vi "html Table.vi"(9 "Rows cnt":u32, 10 "Table Header":string, 11 "In String Table":string[][](array[string])) -> (3 "html string out":string)   [LabVIEW 2018]
panel:
  # "HTML TABLE REPORT GENERATION"
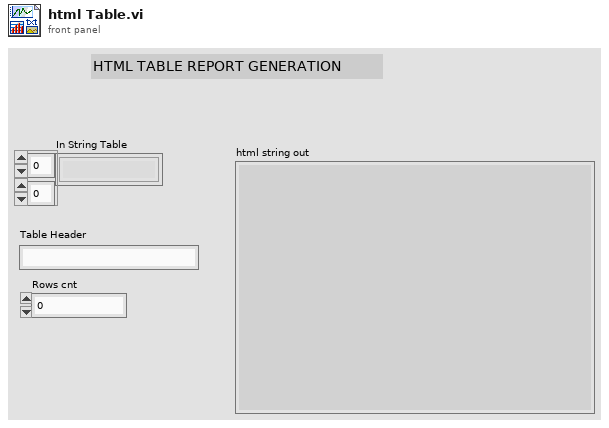
[diagram p1: front panel]
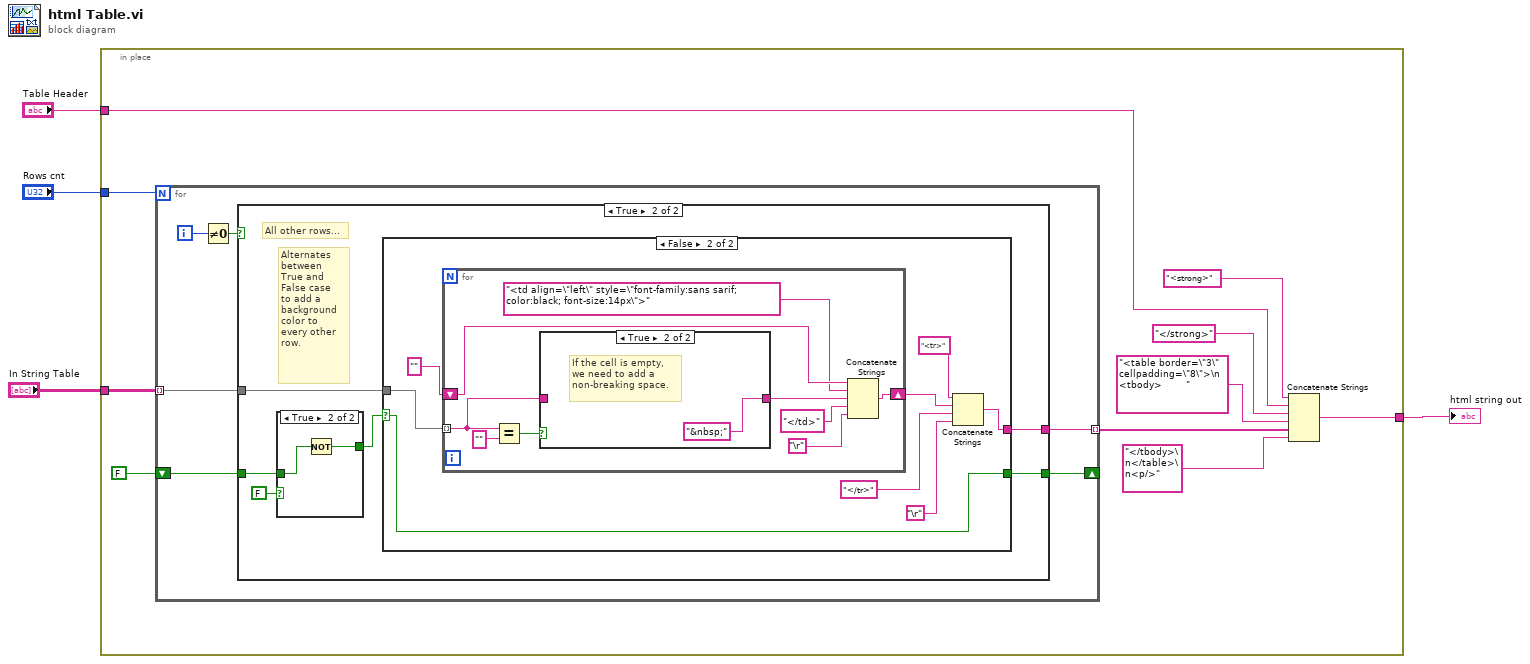
[diagram p0: block diagram]
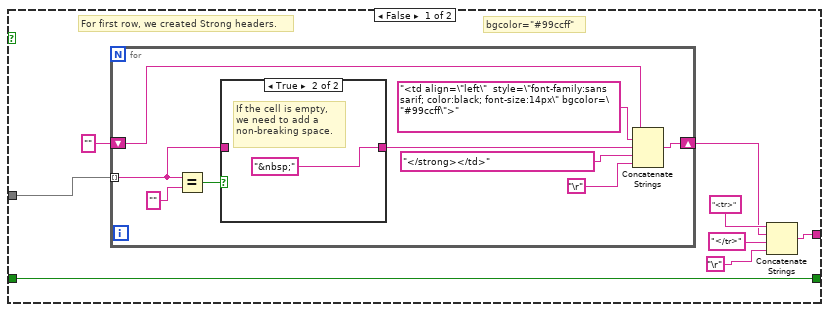
[diagram p2: hidden frame]
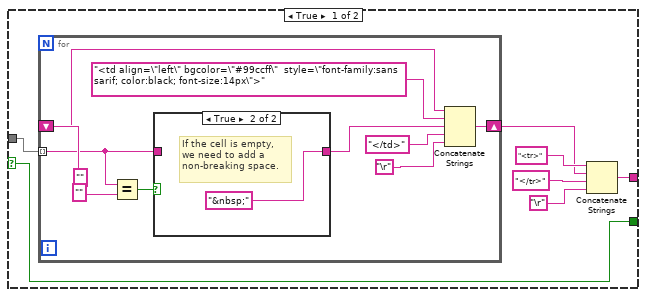
[diagram p5: hidden frame]
diagram:
  n1 = in-place {
    in-place-border: "In String Table" -> [w14]
    in-place-border: "Rows cnt" -> [w12]
    in-place-border: [w8] -> w2
    in-place-border: "Table Header" -> [w6]
    n2 = for {
      N: w12 -> [_]
      tunnel: w14 -> [w20] mode=indexing
      tunnel: [w19] -> w9 mode=indexing
      shift-right: [w15] -> _
      shift-left: FALSE -> [w18]
      i -> [w16]
      n3 = Not Equal To 0?(x=w16) -> (x != 0?=w17:bool)
      n4 = case shown="True" w17 {
        tunnel: w20 -> [w27 w45]
        tunnel: [w23 w44] -> w19
        tunnel: w18 -> [w22 w41]
        tunnel: [w22 w43] -> w15
        frame False {
          # "bgcolor=\"#99ccff\""
          # "For first row, we created Strong headers."
          n5 = for {
            shift-right: [w35] -> w25
            shift-left: "" -> [w34]
            tunnel: w27 -> [w31] mode=indexing
            n6 = Equal?(x=w31, y="") -> (x = y?=w33:bool)
            n7 = case shown="True" w33 {
              tunnel: [w38 "&nbsp;"] -> w32
              tunnel: w31 -> [w38 _]
              frame False {
              }
              frame True {
                # "If the cell is empty, \nwe need to add a \nnon-breaking space."
              }
            }
            n8 = Concatenate Strings(w34, "<td align=\"left\"  style=\"font-family:sans sarif; color:black; font-size:14px\" bgcolor=\"#99ccff\">", w32, "</strong></td>", "\r") -> (w35:string)
          }
          n9 = Concatenate Strings("<tr>", w25, "</tr>", "\r") -> (w23:string)
        }
        frame True {
          # "Alternates \nbetween \nTrue and \nFalse case\nto add a \nbackground \ncolor to \nevery other \nrow."
          # "All other rows..."
          n10 = case shown="True" FALSE {
            tunnel: [w46 w48] -> w42
            tunnel: w41 -> [w46 w47]
            frame False {
            }
            frame True {
              n11 = Not(x=w47) -> (.not. x?=w48:bool)
            }
          }
          n12 = case shown="False" w42 {
            selector: w42 -> [w50 w70]
            tunnel: [w52 w72] -> w44
            tunnel: w45 -> [w51 w71]
            tunnel: [w50 w70] -> w43
            frame True {
              n13 = for {
                tunnel: w51 -> [w59] mode=indexing
                shift-right: [w64] -> w53
                shift-left: "" -> [w63]
                n14 = Equal?(x=w59, y="") -> (x = y?=w62:bool)
                n15 = case shown="True" w62 {
                  tunnel: [w66 "&nbsp;"] -> w60
                  tunnel: w59 -> [w66 _]
                  frame False {
                  }
                  frame True {
                    # "If the cell is empty, \nwe need to add a \nnon-breaking space."
                  }
                }
                n16 = Concatenate Strings(w63, "<td align=\"left\" bgcolor=\"#99ccff\"  style=\"font-family:sans sarif; color:black; font-size:14px\">", w60, "</td>", "\r") -> (w64:string)
              }
              n17 = Concatenate Strings("<tr>", w53, "</tr>", "\r") -> (w52:string)
            }
            frame False {
              n18 = for {
                tunnel: w71 -> [w78] mode=indexing
                shift-right: [w83] -> w73
                shift-left: "" -> [w82]
                n19 = Equal?(x=w78, y="") -> (x = y?=w81:bool)
                n20 = case shown="True" w81 {
                  tunnel: [w85 "&nbsp;"] -> w79
                  tunnel: w78 -> [w85 _]
                  frame False {
                  }
                  frame True {
                    # "If the cell is empty, \nwe need to add a \nnon-breaking space."
                  }
                }
                n21 = Concatenate Strings(w82, "<td align=\"left\" style=\"font-family:sans sarif; color:black; font-size:14px\">", w79, "</td>", "\r") -> (w83:string)
              }
              n22 = Concatenate Strings("<tr>", w73, "</tr>", "\r") -> (w72:string)
            }
          }
        }
      }
    }
    n23 = Concatenate Strings("<strong>", w6, "</strong>", "<table border=\"3\" cellpadding=\"8\">\n    <tbody>        " ("Table Headers"), w9, "</tbody>\n</table>\n<p/>") -> (w8:string)
  }
  "html string out" <- w2
